vi "TestDynamixel.vi"() -> ()   [LabVIEW 2013]
uses:
  Data/TypeDefs/Sail Set Suggestions.ctl
  Data/TypeDefs/Rudder Set Suggestions.ctl
  Data/TypeDefs/MotorSetup.ctl
  Data/TypeDefs/DynamixelSetupInfo.ctl
  Data/TypeDefs/HardwareOnline.ctl
  <instrlib>/Dynamixel Motor/Dynamixel Motor.lvlib
panel:
  out "Dynamixel positions":dbl[](array[numeric])
  out "Initial Hardware Setup":T1
  out "Think Heartbeat":bool
  out "Sense Heartbeat":bool
  out "Act Heartbeat":bool
  out "Current Motor Setup":T2
  in  "Rudder Position Notifier":T4 min=-1.0 max=1.0 scale=1.0..-1.0
  in  "Sail Positions Notifier":T5 {"MainSailSuggestion" min=0.0 max=1.0; "JibSailSuggestion" min=0.0 max=1.0}
  out "Motors IDs Found":u8[](array[numeric])
  in  "stop":bool
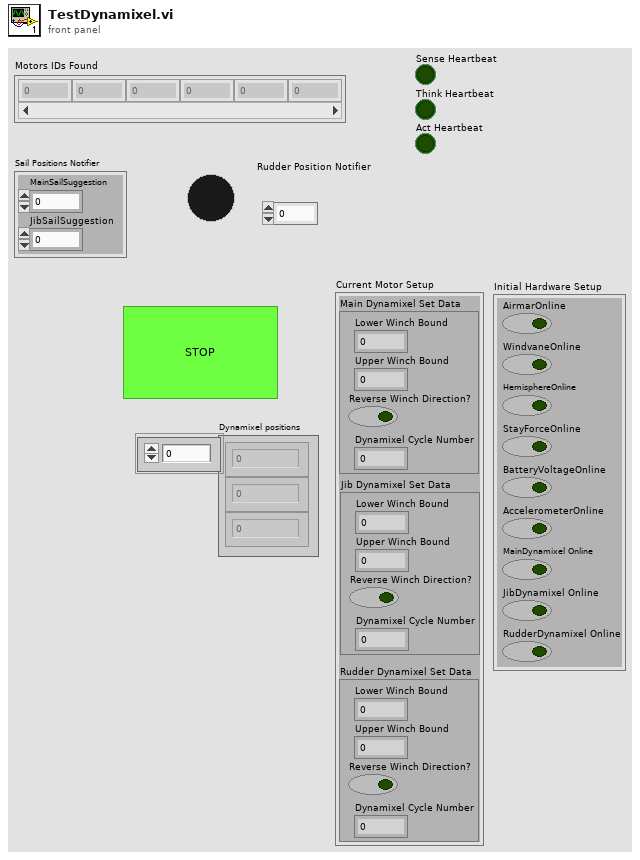
[diagram p1: front panel]
types:
  T1 = typedef "HardwareOnline.ctl" = cluster{"AirmarOnline":bool, "WindvaneOnline":bool, "HemisphereOnline":bool, "StayForceOnline":bool, "BatteryVoltageOnline":bool, "AccelerometerOnline":bool, "MainDynamixel Online":bool, "JibDynamixel Online":bool, "RudderDynamixel Online":bool}
  T2 = typedef "MotorSetup.ctl" = cluster{"Main Dynamixel Set Data":T3, "Rudder Dynamixel Set Data":T3, "Jib Dynamixel Set Data":T3}
  T3 = typedef "DynamixelSetupInfo.ctl" = cluster{"Lower Winch Bound":dbl, "Upper Winch Bound":dbl, "Reverse Winch Direction?":bool, "Dynamixel Cycle Number":i32}
  T4 = typedef "Rudder Set Suggestions.ctl" = dbl
  T5 = typedef "Sail Set Suggestions.ctl" = cluster{"MainSailSuggestion":dbl, "JibSailSuggestion":dbl}
  T6 = enum16{"Blackbody Radiation", "Little boats", "Simulation", "Damn Yankee"}
  T7 = typedef "Notifiers.ctl" = cluster{"BoatSpeed":refnum<notifier>, "WindSpeed":refnum<notifier>, "MissionCheckOff":refnum<notifier>, "EStop":refnum<notifier>, "SpeedOverWater":refnum<notifier>, "BoatDirection":refnum<notifier>, "Luffing":refnum<notifier>, "RudderForce":refnum<notifier>, "BatteryVoltage":refnum<notifier>, "StayForces":refnum<notifier>, "BoatLocation":refnum<notifier>, "Pitch":refnum<notifier>, "Roll":refnum<notifier>, "RateOfTurn":refnum<notifier>, "RelWindDirection":refnum<notifier>, "SailPositions":refnum<notifier>, "RudderPosition":refnum<notifier>, "IronsRange":refnum<notifier>, "AbsWindDirection":refnum<notifier>, "OverrideInformation":refnum<notifier>, "DynamixelTorques":refnum<notifier>, "MotorSetup":refnum<notifier>, "Airmar Status":refnum<notifier>, "HardwareOnline?":refnum<notifier>, "AcutalSimSialPositions":refnum<notifier>}
  T8 = typedef "GPS-Compass Queue Cluster.ctl" = cluster{"BoatLocation Queue":refnum<queue>, "BoatDirection Queue":refnum<queue>, "BoatSpeed Queue":refnum<queue>, "RateOfTurn Queue":refnum<queue>, "Pitch Queue":refnum<queue>, "Roll Queue":refnum<queue>}
  T9 = typedef "WindData Queue Cluster.ctl" = cluster{"RelWindDirection Queue":refnum<queue>, "WindSpeed Queue":refnum<queue>, "AbsWindDirection Queue":refnum<queue>}
  T10 = cluster{"Shroud Queue":refnum<queue>, "Battery Voltage Queue":refnum<queue>, "Accelerometer Queue":refnum<queue>, "AirmarGPS-Compass Queue Cluster":T8, "Hemisphere Queue Cluster":T8, "Airmar Wind Queue Cluster":T9, "Wind Vane Queue Cluster":T9, "Little Boat Queues":cluster{"Heading Queue":refnum<queue>, "Location Queue":refnum<queue>, "Wind Speed Queue":refnum<queue>, "Tilt Queue":refnum<queue>, "Wind Direction Queue":refnum<queue>}, "DynamixelTorque Queue":refnum<queue>, "DynamixelPosition Queue":refnum<queue>}
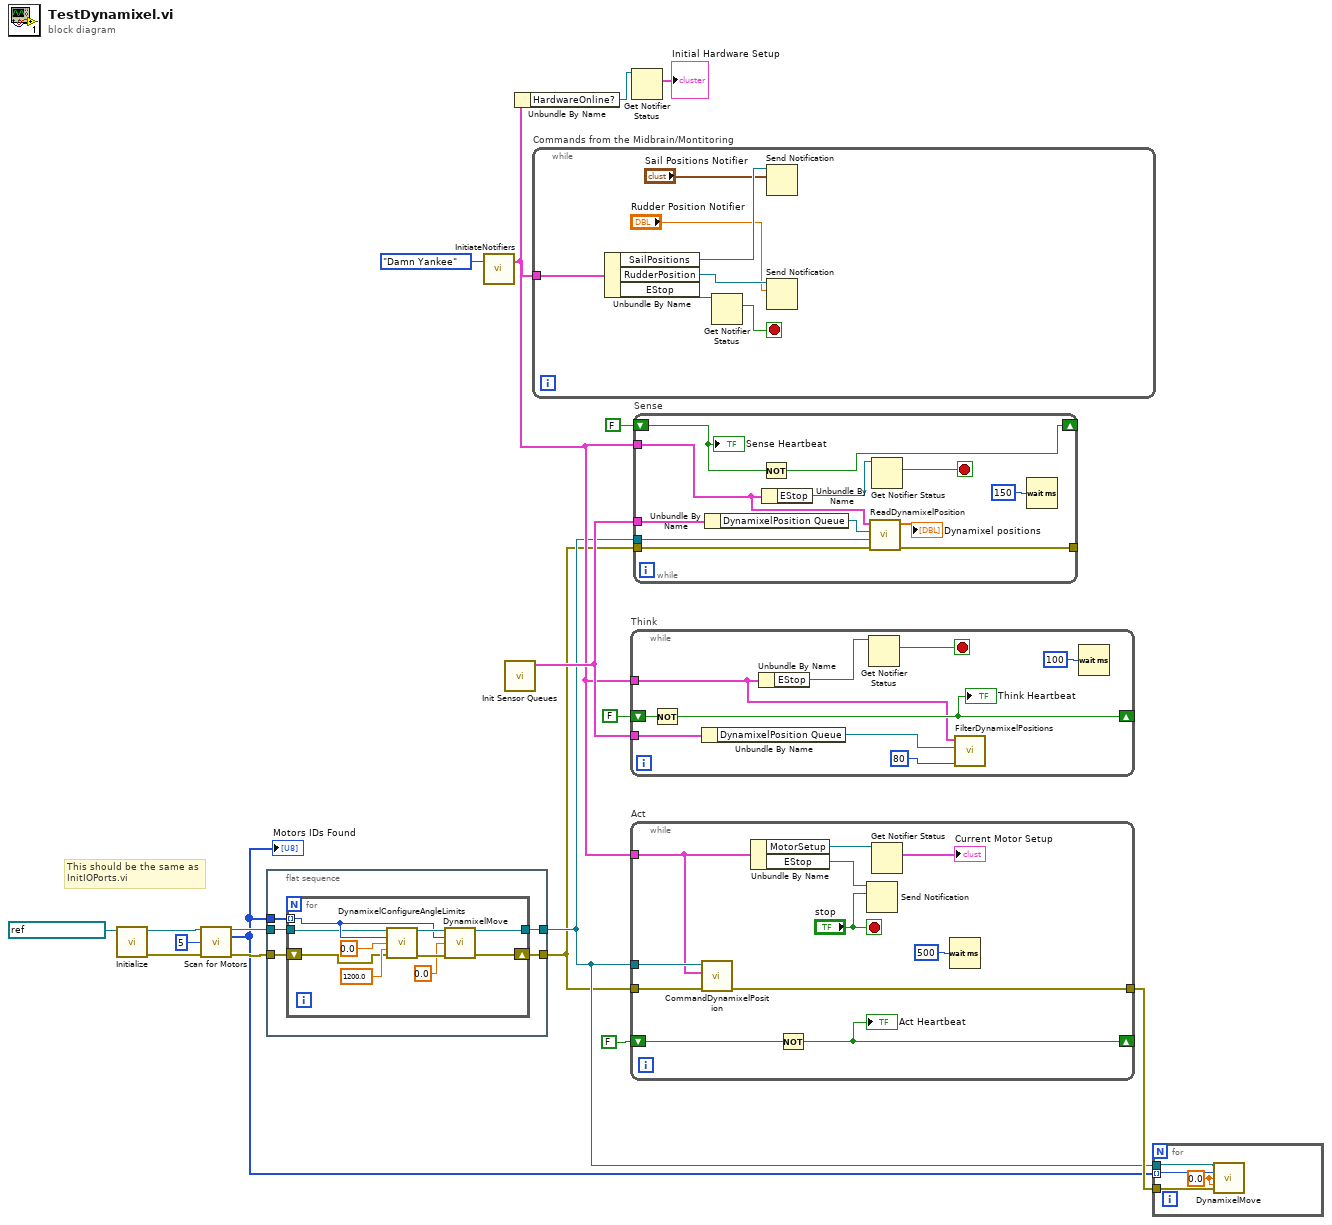
[diagram p0: block diagram]
diagram:
  # "This should be the same as InitIOPorts.vi"
  n1 = call <instrlib>:"Initialize.vi"("VISA resource name"=refnum<visa-resource-name> "ASRL3::INSTR") -> ("error out"=w15:errorcluster, "VISA resource name out"=w16:refnum<visa-resource-name>)  [unwired: 9 in]
  n2 = call <instrlib>:"Scan for Motors.vi"("VISA resource name"=w16, "Ending ID (253)"=u8 5, "error in (no error)"=w15) -> ("VISA resource name out"=w5:refnum<visa-resource-name>, "Motors IDs Found"=w1:u8[], "error out"=w3:errorcluster)  [unwired: 10 in]
  "Motors IDs Found" <- w1
  n3 = flat-sequence {
    tunnel: w5 -> [w21]
    tunnel: [w20] -> w4
    tunnel: w3 -> [w23]
    tunnel: [w22] -> w2
    tunnel: w1 -> [w19]
    frame #0 {
      n4 = for {
        shift-right: [w24] -> w22
        shift-left: w23 -> [w28]
        tunnel: w21 -> [w25]
        tunnel: [w26] -> w20
        tunnel: w19 -> [w29] mode=indexing
        n5 = call "DynamixelConfigureAngleLimits.vi"("VISA resource name"=w25, "Motor ID (0)"=w29, "Clockwise Angle Limit (0 deg)"=0.0, "Counter-Clockwise Angle Limit (300 deg)"=1200.0, "error in (no error)"=w28) -> ("VISA resource name out"=w32:refnum<visa-resource-name>, "error out"=w33:errorcluster)  [unwired: 9 in]
        n6 = call "DynamixelMove.vi"("VISA resource name"=w32, "Motor ID (0)"=w29, "Goal Position (150 deg)"=0.0, "error in (no error)"=w33) -> ("VISA resource name out"=w26:refnum<visa-resource-name>, "error out"=w24:errorcluster)  [unwired: 10 in]
      }
    }
  }
  n7 = call "InitiateNotifiers.vi"("Boat Type"=T6."Damn Yankee") -> ("NotifierReferences"=w9:T7)  [unwired: 1 in, 1 out]
  n8 = call "Init Sensor Queues.vi"() -> ("output cluster"=w13:T10)  [unwired: 11 in]
  n9 = Unbundle By Name(w9) -> ("HardwareOnline?"=w8:refnum<notifier>)
  n10 = while "Commands from the Midbrain/Montitoring" {
    tunnel: w9 -> [w40]
    stop <- w38 stop-if-true
    n11 = Unbundle By Name(w40) -> ("SailPositions"=w37:refnum<notifier>, "RudderPosition"=w36:refnum<notifier>, "EStop"=w39:refnum<notifier>)
    n12 = Get Notifier Status(notifier=w39) -> (current notification=w38:bool)  [unwired: 1 in, 4 out]
    n13 = Send Notification(notification="Sail Positions Notifier", notifier=w37) -> ()  [unwired: 1 in, 2 out]
    n14 = Send Notification(notification="Rudder Position Notifier", notifier=w36) -> ()  [unwired: 1 in, 2 out]
  }
  n15 = while "Think" {
    tunnel: w9 -> [w41]
    tunnel: w13 -> [w49]
    shift-right: [w43] -> _
    shift-left: FALSE -> [w44]
    stop <- w45 stop-if-true
    n16 = Not(x=w44) -> (.not. x?=w43:bool)
    "Think Heartbeat" <- w43
    n17 = Unbundle By Name(w49) -> ("DynamixelPosition Queue"=w48:refnum<queue>)
    n18 = Unbundle By Name(w41) -> ("EStop"=w46:refnum<notifier>)
    n19 = Get Notifier Status(notifier=w46) -> (current notification=w45:bool)  [unwired: 1 in, 4 out]
    n20 = call "FilterDynamixelPositions.vi"("Queue timeout (ms)"=80, "DynamixelPosition Queue"=w48, "NotifierReff"=w41) -> ()  [unwired: 9 in]
    n21 = Wait (ms)(milliseconds to wait=u32 100) -> ()  [unwired: 1 out]
  }
  n22 = while "Act" {
    tunnel: w4 -> [w59]
    tunnel: w2 -> [w58]
    tunnel: w9 -> [w57]
    tunnel: [w52] -> w6
    shift-right: [w50] -> _
    shift-left: FALSE -> [w51]
    stop <- "stop" stop-if-true
    n23 = call "CommandDynamixelPosition.vi"("error in"=w58, "NotifierReff"=w57, "VISA resource name"=w59) -> ("Error out"=w52:errorcluster)  [unwired: 8 in]
    n24 = Unbundle By Name(w57) -> ("MotorSetup"=w54:refnum<notifier>, "EStop"=w56:refnum<notifier>)
    n25 = Not(x=w51) -> (.not. x?=w50:bool)
    "Act Heartbeat" <- w50
    n26 = Send Notification(notification="stop", notifier=w56) -> ()  [unwired: 1 in, 2 out]
    n27 = Get Notifier Status(notifier=w54) -> (current notification=→"Current Motor Setup":T2)  [unwired: 1 in, 4 out]
    n28 = Wait (ms)(milliseconds to wait=u32 500) -> ()  [unwired: 1 out]
  }
  n29 = Get Notifier Status(notifier=w8) -> (current notification=→"Initial Hardware Setup":T1)  [unwired: 1 in, 4 out]
  n30 = while "Sense" {
    tunnel: w13 -> [w72]
    tunnel: w9 -> [w62]
    tunnel: w4 -> [w70]
    tunnel: w2 -> [w69]
    tunnel: [w68] -> _
    shift-right: [w65] -> _
    shift-left: FALSE -> [w64]
    stop <- w66 stop-if-true
    n31 = Unbundle By Name(w72) -> ("DynamixelPosition Queue"=w71:refnum<queue>)
    n32 = Not(x=w64) -> (.not. x?=w65:bool)
    n33 = Unbundle By Name(w62) -> ("EStop"=w67:refnum<notifier>)
    n34 = call "ReadDynamixelPosition.vi"("error in (no error)"=w69, "VISA resource name"=w70, "DynamixelPositions Queue"=w71, "Notifier References"=w62) -> ("error out"=w68:errorcluster, "Dynamixel positions"=→"Dynamixel positions":dbl[])  [unwired: 6 in]
    n35 = Get Notifier Status(notifier=w67) -> (current notification=w66:bool)  [unwired: 1 in, 4 out]
    n36 = Wait (ms)(milliseconds to wait=u32 150) -> ()  [unwired: 1 out]
    "Sense Heartbeat" <- w64
  }
  n37 = for {
    tunnel: w4 -> [w76]
    tunnel: w6 -> [w75]
    tunnel: w1 -> [w74] mode=indexing
    w73 = 0.0 ("Goal Position (150 deg)")
    n38 = call "DynamixelMove.vi"("VISA resource name"=w76, "Motor ID (0)"=w74, "Goal Position (150 deg)"=w73, "Goal Speed (RPM)"=w73, "error in (no error)"=w75) -> ()  [unwired: 9 in, 2 out]
  }
